vi "OCR Example DNN.vi"() -> ()   [LabVIEW 2020, in "examples.lvlib"]
uses:
  examples.lvlib
  feature_detection/Text Detector/Detection.ctl
  common/Quad Corners.ctl
  common/Image Point (Float).ctl
  image/ARGB Colour.ctl
  common/Image Size (Integer).ctl
  common/Image Point (Integer).ctl
  feature_detection/Text Detector/Text Detector.lvclass/Text Detector.ctl
  feature_detection/Text Recognizer/Text Recognizer.lvclass/Text Recognizer.ctl
  image/New Image (ARGB Preallocated).vi
  image/Warp Perspective (ARGB).vi
  image/Draw Poly Lines (ARGB).vi
  image/Draw Image to Picture (ARGB).vi
  image/New Image (ARGB Preallocated).vi/3321fa97-f432-4e1e-8db9-a0df79aed21b.vi
  image/ARGB Colour to U32 Pixel Value.vi
  feature_detection/Text Detector/Build Model Data Cluster.vi
  image/Draw Text (ARGB).vi/0015c4fc-6a12-4f82-815b-6c2f827f408b.vi
  feature_detection/Text Detector/Detect Text (ARGB).vi/eed31af3-93fd-418d-8fe9-3dec6e1d7c5b.vi
  image/Warp Perspective (ARGB).vi/2e2371c9-0103-42e0-a64c-538b92d2b12b.vi
  feature_detection/Text Recognizer/Recognize Text (ARGB).vi/2becd383-3adf-4b47-81eb-e38e0ef2f6e5.vi
  image/Draw Poly Lines (ARGB).vi/f4fe866f-059f-471d-887d-2797bd4b3b13.vi
  image/Draw Image to Picture (ARGB).vi/8cd07b1b-062e-4fe4-9e87-2eb3dc89fe0e.vi
  feature_detection/Text Detector/Path to String Path.vi
  image/Warp Perspective (ARGB).vi/2e2371c9-0103-42e0-a64c-538b92d2b12b.vi/0c263cf4-9042-4d44-b92e-dafa676e1650.vi
  <vilib>/Utility/error.llb/Error Cluster From Error Code.vi
  <vilib>/Analysis/Matrix/Numeric/Conversions/Array To Matrix.vi
  <vilib>/Analysis/Matrix/Numeric/Conversions/Array To Matrix - RA2.vi
  feature_detection/Text Detector/Text Detector.lvclass
  image/image.lvlib
  feature_detection/Text Recognizer/Text Recognizer.lvclass
  common/common.lvlib
panel:
  in  "Model":enum16{"EAST", "DB Net (PP OCRv3)"}(ring)
  out "Text":string[](array[string])
  out "Detections":T1[](array[typedef])
  out "Output":picture
  # "See Block Diagram for Instructions on Downloading Model-Files"
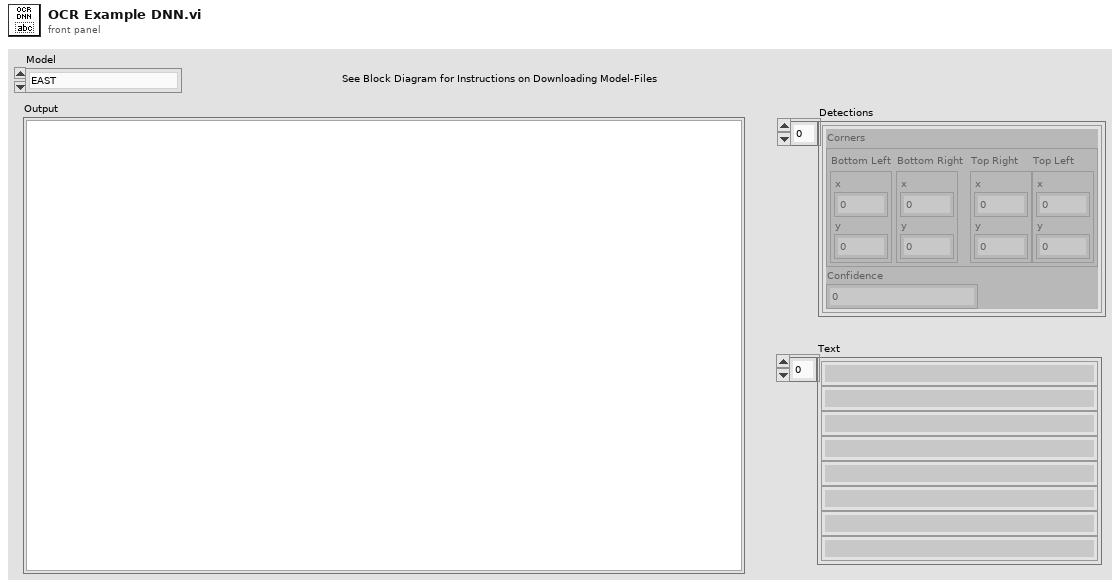
[diagram p1: front panel]
types:
  T1 = typedef "feature_detection.lvlib/Text Detector.lvclass/Detection.ctl" = cluster{"Corners":T2, "Confidence":sgl}
  T2 = typedef "common.lvlib/Quad Corners.ctl" = cluster{"Bottom Left":T3, "Bottom Right":T3, "Top Right":T3, "Top Left":T3}
  T3 = typedef "common.lvlib/Image Point (Float).ctl" = cluster{"x":dbl, "y":dbl}
  T4 = typedef "image.lvlib/ARGB Colour.ctl" = cluster{"Alpha":u8, "RGB":u32}
  T5 = typedef "common.lvlib/Image Point (Integer).ctl" = cluster{"x":i32, "y":i32}
  T6 = typedef "common.lvlib/Image Size (Integer).ctl" = cluster{"Width":u16, "Height":u16}
  T7 = typedef "feature_detection.lvlib/Text Detector.lvclass/Model.ctl" = cluster{"Model Data":path, "Model Config":path, "Image Size":T6, "Mean":T8, "Scale":dbl, "Expects RGB Channel Order":bool}
  T8 = typedef "common.lvlib/Object Point (Float).ctl" = cluster{"x":dbl, "y":dbl, "z":dbl}
  T9 = typedef "feature_detection.lvlib/Text Recognizer.lvclass/Model.ctl" = cluster{"Model Data":path, "Model Config":path, "Vocabulary":string, "Mode":T10, "Image Size":T6, "Mean":T8, "Scale":dbl, "Expects RGB Channel Order":bool}
  T10 = typedef "feature_detection.lvlib/Text Recognizer.lvclass/Mode.ctl" = enum8{"CTC-greedy", "CTC-prefix-beam-search"}
  T11 = typedef "image.lvlib/ARGB Image.ctl" = refnum<data-value>
  T12 = typedef "NI_Matrix.lvlib/RealMatrix.ctl" = dbl[][]
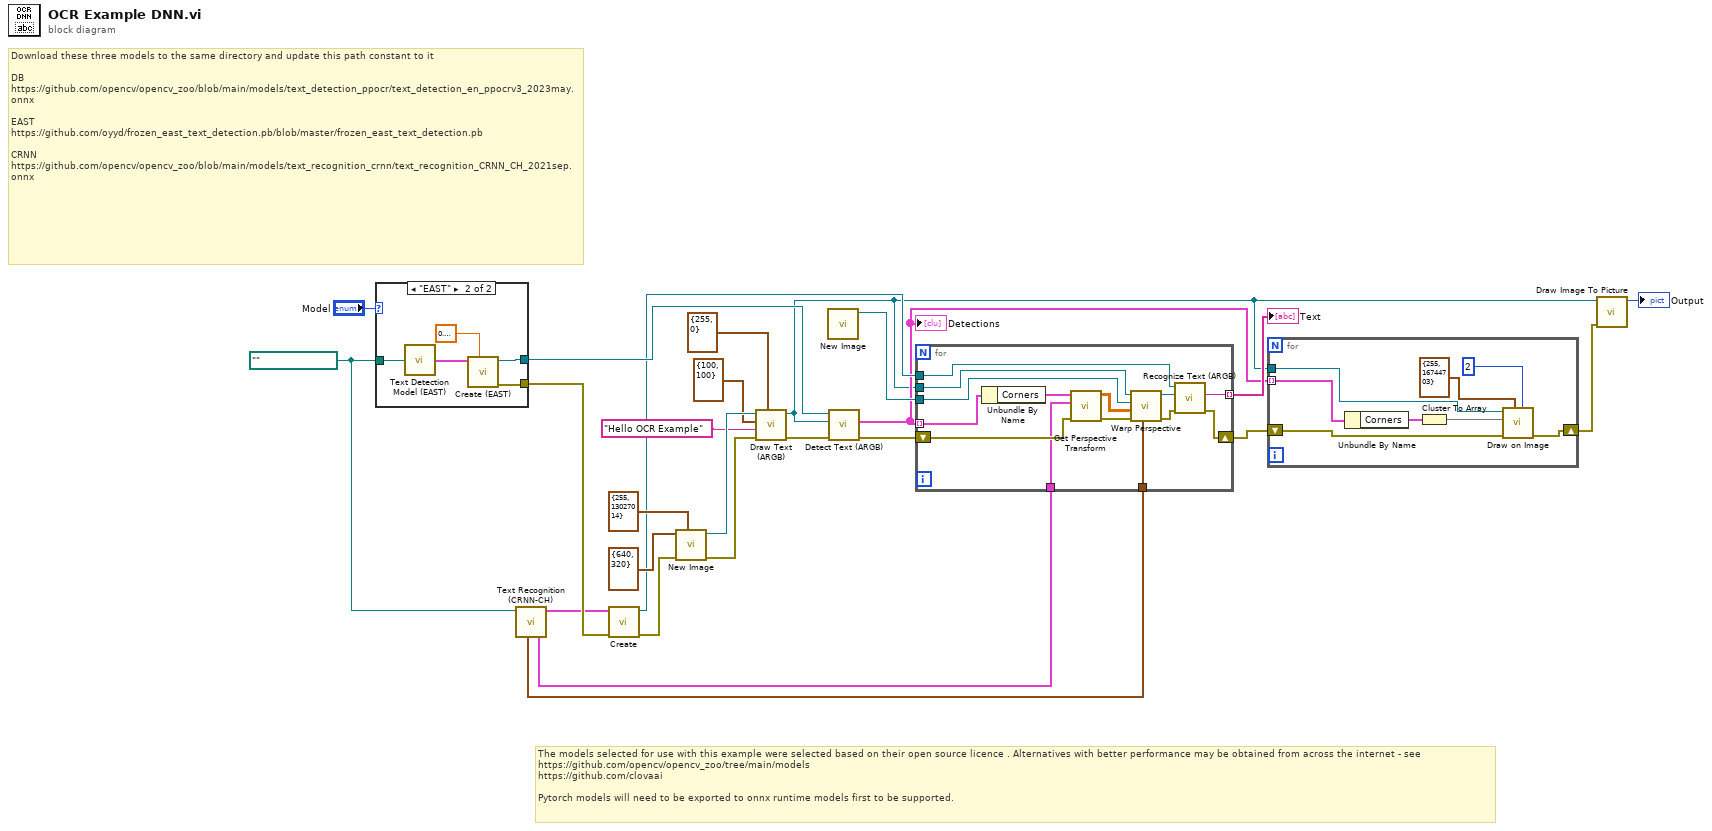
[diagram p0: block diagram]
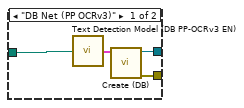
[diagram p2: hidden frame]
diagram:
  w1 = path "" ("Model Path Directory (Default: Relative to This VI)")
  # "Download these three models to the same directory and update this path constant to it\n\nDB\nhttps://github.com/opencv/opencv_zoo/blob/main/models/text_detection_ppocr/text_detection_en_ppocrv3_2023may.onnx\n\nEAST\nhttps://github.com/oyyd/frozen_east_text_detection.pb/blob/master/frozen_east_text_detection.pb\n\nCRNN\nhttps://github.com/opencv/opencv_zoo/blob/main/models/text_recognition_crnn/text_recognition_CRNN_CH_2021sep.onnx"
  # "The models selected for use with this example were selected based on their open source licence . Alternatives with better performance may be obtained from across the internet - see \nhttps://github.com/opencv/opencv_zoo/tree/main/models\nhttps://github.com/clovaai\n\nPytorch models will need to be exported to onnx runtime models first to be supported."
  n1 = case shown="\"EAST\"" "Model" {
    tunnel: [w28 w34] -> w23
    tunnel: [w27 w31] -> w5
    tunnel: w1 -> [w26 w30]
    frame "DB Net (PP OCRv3)" {
      n2 = call "Text Detection Model (DB PP-OCRv3 EN).vi"("Model Path Directory (Default: Relative to This VI)"=w26) -> ("Text Detection Model (DB)"=w29:T7)
      n3 = call "Create (DB).vi"("Model"=w29) -> ("error out"=w27:errorcluster, "Text Detector"=w28:refnum<class "Text Detector.lvclass">)  [unwired: 9 in]
    }
    frame "EAST" {
      n4 = call "Text Detection Model (EAST).vi"("Model Path Directory (Default: Relative to This VI)"=w30) -> ("Text Detection Model (EAST)"=w32:T7)
      n5 = call "Create (EAST).vi"("Confidence Threshold (Default: 0.5)"=sgl 0.3 ("conf_threshold"), "Model"=w32) -> ("error out"=w31:errorcluster, "Text Detector"=w34:refnum<class "Text Detector.lvclass">)  [unwired: 8 in]
    }
  }
  n6 = call "Text Recognition (CRNN-CH).vi"("Model Path Directory (Default: Relative to This VI)"=w1) -> ("Text Recognizer Model"=w4:T9, "Target Corners"=w3:T2, "Target Size"=w2:T6)  [unwired: 8 in]
  n7 = call "Create.vi"("error in (no error)"=w5, "Model"=w4) -> ("error out"=w7:errorcluster, "Text Recognizer"=w12:refnum<class "Text Recognizer.lvclass">)  [unwired: 8 in]
  n8 = call-poly "New Image.vi"("Colour (Default: Black)"=T4 {"Alpha"=255, "RGB"=13027014}, "error in (no error)"=w7, "Preallocated Image Size (Default: 0,0)"=T6 {"Width"=640, "Height"=320}) -> ("error out"=w20:errorcluster, "ARGB Image"=w21:T11)  [unwired: 7 in]
  n9 = call "Draw Text (ARGB).vi"("ARGB Colour"=T4 {"Alpha"=255, "RGB"=0}, "error in (no error)"=w20, "Text"="Hello OCR Example", "Origin"=T5 {"x"=100, "y"=100}, "ARGB Image in"=w21) -> ("error out"=w8:errorcluster, "ARGB Image"=w6:T11)  [unwired: 5 in]
  n10 = call-poly "New Image.vi"() -> ("ARGB Image"=w13:T11)  [unwired: 10 in, 1 out]
  n11 = call "Detect Text (ARGB).vi"("error in (no error)"=w8, "ARGB Image in"=w6, "Text Detector in"=w23) -> ("error out"=w14:errorcluster, "Detections"=w10:T1[])  [unwired: 6 in, 1 out]
  "Detections" <- w10
  n12 = for {
    tunnel: w10 -> [w48] mode=indexing
    shift-right: [w37] -> w9
    shift-left: w14 -> [w46]
    tunnel: w13 -> [w45]
    tunnel: w12 -> [w42]
    tunnel: [w40] -> w11 mode=indexing
    tunnel: w6 -> [w38]
    tunnel: w3 -> [w36]
    tunnel: w2 -> [w35]
    n13 = Unbundle By Name(w48) -> ("Corners"=w47:T2)
    n14 = call "Get Perspective Transform.vi"("error in (no error)"=w46, "To"=w36, "From"=w47) -> ("error out"=w43:errorcluster, "3x3 Warp Matrix"=w44:T12)  [unwired: 7 in]
    n15 = call-poly "Warp Perspective.vi"("Required Destination Size"=w35, "error in (no error)"=w43, "3x3 Warp Matrix"=w44, "ARGB Destination Image in"=w45, "ARGB Source Image in"=w38) -> ("error out"=w41:errorcluster, "ARGB  Destination Image"=w39:T11)  [unwired: 5 in]
    n16 = call "Recognize Text (ARGB).vi"("error in (no error)"=w41, "ARGB Image in"=w39, "Text Recognizer in"=w42) -> ("error out"=w37:errorcluster, "Recognition"=w40:string)  [unwired: 6 in, 1 out]
  }
  "Text" <- w11
  n17 = for {
    tunnel: w10 -> [w54] mode=indexing
    shift-right: [w55] -> w24
    shift-left: w9 -> [w56]
    tunnel: w6 -> [w49]
    n18 = Unbundle By Name(w54) -> ("Corners"=w53:T2)
    n19 = Cluster To Array(cluster=w53) -> (array=w52:T3[])
    n20 = call-poly "Draw on Image.vi"("Thickness (Default: 1)"=2, "ARGB Colour"=T4 {"Alpha"=255, "RGB"=16744703}, "error in (no error)"=w56, "Points"=w52, "ARGB Image in"=w49) -> ("error out"=w55:errorcluster)  [unwired: 5 in, 1 out]
  }
  n21 = call-poly "Draw Image To Picture.vi"("error in (no error)"=w24, "ARGB Image Source in"=w6) -> ("Picture"=→"Output":picture)  [unwired: 8 in, 1 out]
